vi "Get Baud Rate.vi"(8 "error in":errorcluster, 11 "IHas Baudrate in":refnum<class "PCAN Base Strategy.lvclass">) -> (0 "error out":errorcluster, 2 "Baud Rate":u32, 3 "IHas Baudrate out":refnum<class "PCAN Base Strategy.lvclass">)   [LabVIEW 2024, in "PCAN Base Strategy.lvclass"]
uses:
  PCAN Base Strategy.lvclass
  PCAN Base Strategy.lvclass/PCAN Base Strategy.ctl
  Source/Interfaces/IConfiguration/IConfiguration.lvclass
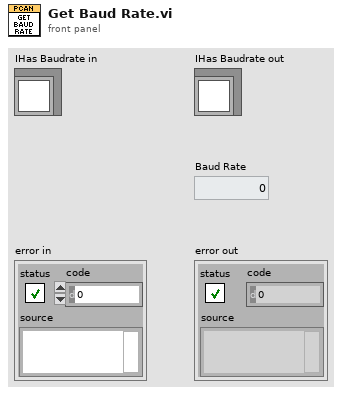
[diagram p1: front panel]
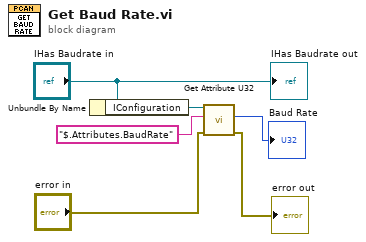
[diagram p0: block diagram]
diagram:
  n1 = Unbundle By Name("IHas Baudrate in") -> ("IConfiguration"=w5:refnum<class "IConfiguration.lvclass">)
  n2 = call-dynamic "Get Attribute U32.vi"("error in"="error in", "Attribute"="$.Attributes.BaudRate", "IConfiguration in"=w5) -> ("error out"=→"error out":errorcluster, "Value"=→"Baud Rate":u32)  [unwired: 6 in, 1 out]
  "IHas Baudrate out" <- "IHas Baudrate in"
